vi "Untitled 2.vi"() -> ()   [LabVIEW 2020]
uses:
  labview_control/LaoJi/LMMR ASG/ASG Instructions XControl.xctl
  labview_control/LaoJi/NI CTR/NI DAQ Counter.lvlib
  labview_control/LaoJi/LMMR ASG/ASG 8100 Module.lvlib
panel:
  out "System Waveform Chart":u32[](graph)
  out "Sample Array 2":u32[](array[numeric])
  in  "CW seq":T1(xcontrol)=[{"Flags"=[FALSE, FALSE, FALSE, FALSE, FALSE, FALSE, FALSE, FALSE, FALSE, FALSE, FALSE, FALSE, FALSE, FALSE], "Comments"="", "Time"=1e-05, "Loop Config"={"Loop Code"=0, "Number of Loop"=0, "Loop Info"="", "End of Loop"=nan}}, {"Flags"=[FALSE, FALSE, TRUE, FALSE, FALSE, FALSE, FALSE, FALSE, FALSE, FALSE, FALSE, FALSE, FALSE, FALSE], "Comments"="", "Time"=5e-08, "Loop Config"={"Loop Code"=0, "Number of Loop"=0, "Loop Info"="", "End of Loop"=nan}}, {"Flags"=[TRUE, TRUE, FALSE, FALSE, FALSE, FALSE, FALSE, FALSE, FALSE, FALSE, FALSE, FALSE, FALSE, FALSE], "Comments"="", "Time"=0.0005, "Loop Config"={"Loop Code"=0, "Number of Loop"=0, "Loop Info"="", "End of Loop"=nan}}, {"Flags"=[FALSE, FALSE, TRUE, FALSE, FALSE, FALSE, FALSE, FALSE, FALSE, FALSE, FALSE, FALSE, FALSE, FALSE], "Comments"="", "Time"=5e-08, "Loop Config"={"Loop Code"=0, "Number of Loop"=0, "Loop Info"="", "End of Loop"=nan}}, {"Flags"=[FALSE, FALSE, FALSE, FALSE, FALSE, FALSE, FALSE, FALSE, FALSE, FALSE, FALSE, FALSE, FALSE, FALSE], "Comments"="", "Time"=1e-05, "Loop Config"={"Loop Code"=0, "Number of Loop"=0, "Loop Info"="", "End of Loop"=nan}}, {"Flags"=[FALSE, FALSE, TRUE, FALSE, FALSE, FALSE, FALSE, FALSE, FALSE, FALSE, FALSE, FALSE, FALSE, FALSE], "Comments"="", "Time"=5e-08, "Loop Config"={"Loop Code"=0, "Number of Loop"=0, "Loop Info"="", "End of Loop"=nan}}, {"Flags"=[TRUE, FALSE, FALSE, FALSE, FALSE, FALSE, FALSE, FALSE, FALSE, FALSE, FALSE, FALSE, FALSE, FALSE], "Comments"="", "Time"=0.0005, "Loop Config"={"Loop Code"=0, "Number of Loop"=0, "Loop Info"="", "End of Loop"=nan}}, {"Flags"=[FALSE, FALSE, TRUE, FALSE, FALSE, FALSE, FALSE, FALSE, FALSE, FALSE, FALSE, FALSE, FALSE, FALSE], "Comments"="", "Time"=5e-08, "Loop Config"={"Loop Code"=0, "Number of Loop"=0, "Loop Info"="", "End of Loop"=nan}}, {"Flags"=[FALSE, FALSE, FALSE, FALSE, FALSE, FALSE, FALSE, FALSE, FALSE, FALSE, FALSE, FALSE, FALSE, FALSE], "Comments"="", "Time"=1e-05, "Loop Config"={"Loop Code"=0, "Number of Loop"=0, "Loop Info"="", "End of Loop"=nan}}, {"Flags"=[FALSE, FALSE, FALSE, FALSE, FALSE, FALSE, FALSE, FALSE, FALSE, FALSE, FALSE, FALSE, FALSE, FALSE], "Comments"="", "Time"=1e-06, "Loop Config"={"Loop Code"=0, "Number of Loop"=0, "Loop Info"="", "End of Loop"=nan}}]
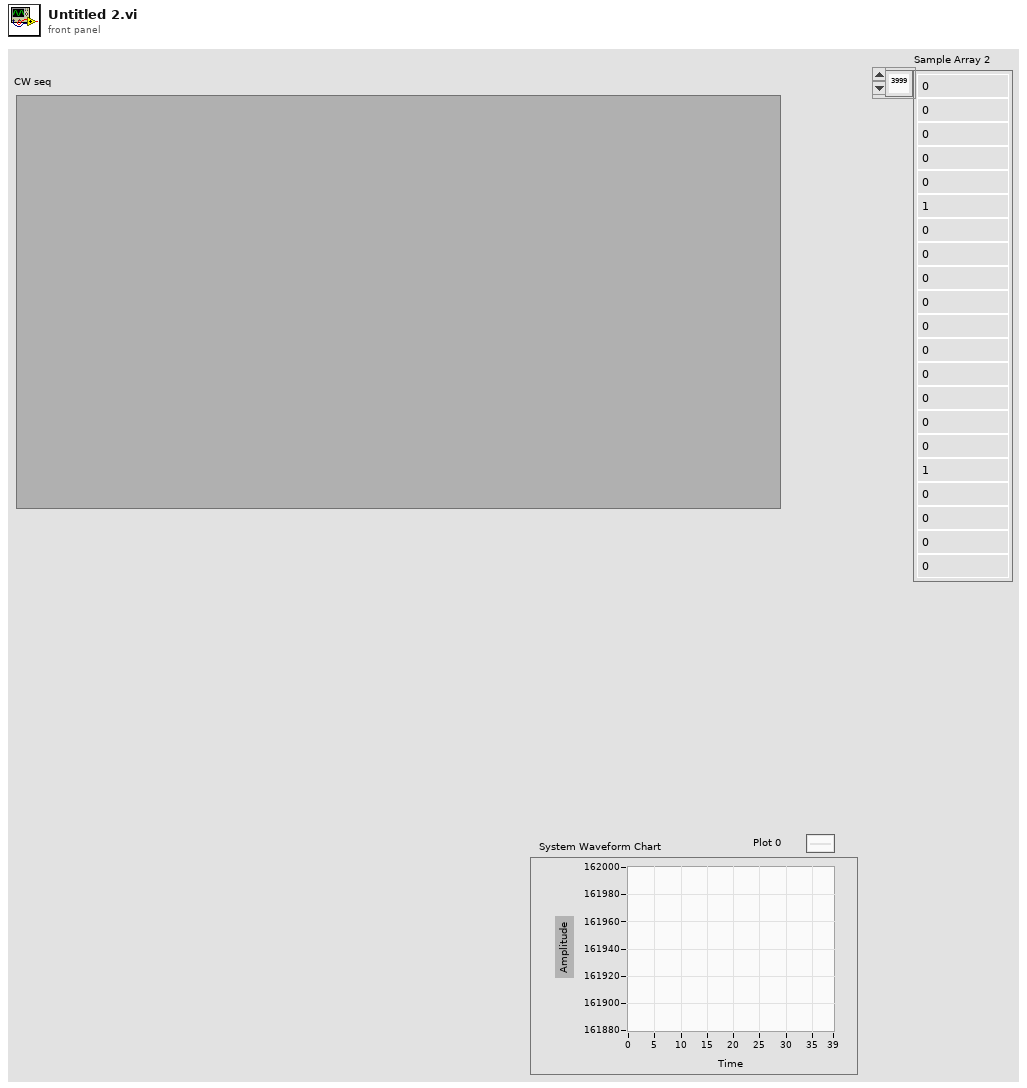
[diagram p1: front panel]
types:
  T1 = cluster{"Flags":bool[], "Comments":string, "Time":dbl, "Loop Config":cluster{"Loop Code":u16, "Number of Loop":i32, "Loop Info":string, "End of Loop":dbl}}[]
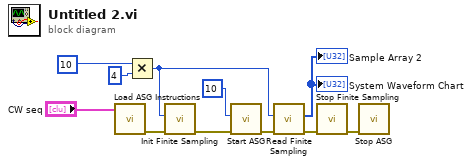
[diagram p0: block diagram]
diagram:
  n1 = call "Load ASG Instructions.vi"("ASG Instructions"="CW seq") -> ("error out"=w11:errorcluster)  [unwired: 10 in]
  n2 = Multiply(x=10, y=4) -> (x*y=w6:i32)
  n3 = call "Init Finite Sampling.vi"("error in (no error)"=w11, "Num of Sample"=w6) -> ("error out"=w10:errorcluster)  [unwired: 9 in]
  n4 = call "Start ASG.vi"("error in (no error)"=w10, "Loop Number"=10) -> ("error out"=w9:errorcluster)  [unwired: 8 in, 1 out]
  n5 = call "Read Finite Sampling.vi"("error in (no error)"=w9, "Samples to Read"=w6) -> ("error out"=w8:errorcluster, "Sample Array"=→"Sample Array 2" →"System Waveform Chart":u32[])  [unwired: 7 in, 1 out]
  n6 = call "Stop Finite Sampling.vi"("error in (no error)"=w8) -> ("error out"=w7:errorcluster)  [unwired: 10 in]
  n7 = call "Stop ASG.vi"("error in (no error)"=w7) -> ()  [unwired: 9 in, 2 out]
